vi "NumberDetector.vi"() -> ()   [LabVIEW 2016]
uses:
  <vilib>/Analysis/3filter.llb/Filter Passband Type.ctl
  <vilib>/myRIO/Instrument Drivers/Onboard Devices/Accelerometer/typedefs/Accelerometer Reference.ctl
  <vilib>/myRIO/Common/Instrument Driver Framework/Utilities/typedefs/myRIO Generic Hardware Reference.ctl
  <vilib>/myRIO/Common/Instrument Driver Framework/Utilities/typedefs/Hardware Version Enum.ctl
  <vilib>/myRIO/Common/Instrument Driver Framework/Utilities/typedefs/myRIO v1.0 Reference.ctl
  <vilib>/myRIO/Common/Instrument Driver Framework/Utilities/typedefs/Generic FPGA Reference.ctl
  <vilib>/myRIO/Common/Instrument Driver Framework/myRIO v1.0/Accelerometer/typedefs/Accelerometer Channels List.ctl
  <vilib>/myRIO/Common/Instrument Driver Framework/myRIO v1.0/Accelerometer/typedefs/Accelerometer Channels Enum.ctl
  <vilib>/userdefined/High Color/nirio_resource_hc.ctl
  <vilib>/myRIO/Common/Instrument Driver Framework/Utilities/vis/Is FPGA Ref Available.vi
  <vilib>/myRIO/Common/Instrument Driver Framework/myRIO v1.0/Accelerometer/vis/myRIO v1.1 Open Accelerometer.vi
  <vilib>/myRIO/Instrument Drivers/Onboard Devices/Accelerometer/vis/Read.vi
  <vilib>/Analysis/baseanly.llb/A x Vector.vi
  <vilib>/myRIO/Common/Instrument Driver Framework/Utilities/vis/Validate Channels.vi
  <vilib>/myRIO/Common/Instrument Driver Framework/myRIO v1.0/Accelerometer/vis/myRIO v1.0 Reserve Accelerometer.vi
  <vilib>/myRIO/Common/Instrument Driver Framework/myRIO v1.0/UART/vis/myRIO v1.0 Close UART.vi
  <vilib>/myRIO/Common/Instrument Driver Framework/myRIO v1.0/Resource Manager/vis/myRIO v1.0 Reserve Channel List.vi
  <vilib>/myRIO/Common/Instrument Driver Framework/myRIO v1.0/Accelerometer/vis/myRIO v1.0 Build MUX Configuration Accelerometer.vi
  <vilib>/myRIO/Common/Instrument Driver Framework/myRIO v1.0/Resource Manager/vis/myRIO v1.0 Reserve Channel.vi
  <vilib>/myRIO/Common/Instrument Driver Framework/myRIO v1.0/Resource Manager/vis/myRIO v1.0 Unreserve Channel.vi
  <vilib>/myRIO/Common/Instrument Driver Framework/myRIO v1.0/Resource Manager/vis/myRIO v1.0 Build Mutex Name.vi
  <vilib>/Utility/VariantDataType/GetNumericInfo.vi
  <vilib>/Utility/error.llb/Error Cluster From Error Code.vi
  <vilib>/myRIO/Common/Instrument Driver Framework/myRIO v1.0/myRIO v1.1 Open.vi
  <vilib>/myRIO/Common/Instrument Driver Framework/myRIO v1.0/Accelerometer/vis/myRIO v1.0 Get Scaling Constant Accelerometer.vi
  <vilib>/myRIO/Common/Instrument Driver Framework/Utilities/vis/IO Manager.vi
  <vilib>/myRIO/Common/Instrument Driver Framework/Utilities/vis/Configuration Manager.vi
  <vilib>/myRIO/Common/Instrument Driver Framework/myRIO v1.0/myRIO v1.0 Close.vi
  <vilib>/myRIO/Common/Instrument Driver Framework/myRIO v1.0/Accelerometer/vis/myRIO v1.0 Read Accelerometer.vi
  <vilib>/myRIO/Common/Instrument Driver Framework/Utilities/vis/FPGA Ref Manager.vi
  <vilib>/myRIO/Common/Instrument Driver Framework/myRIO v1.0/myRIO v1.0 Reset FPGA.vi
  <vilib>/myRIO/Common/Instrument Driver Framework/myRIO v1.0/IRQ/vis/myRIO v1.0 IRQ Info FGV.vi
  <vilib>/myRIO/Common/Instrument Driver Framework/myRIO v1.0/IRQ/vis/myRIO v1.0 Timer IRQ Info FGV.vi
  <vilib>/myRIO/Common/Instrument Driver Framework/myRIO v1.0/IRQ/vis/myRIO v1.0 ISR Agent.vi
  <vilib>/myRIO/Express VI/Onboard Devices/Accelerometer/Accelerometer Express VI.xnode
  <vilib>/myRIO/Instrument Drivers/Onboard Devices/Accelerometer/vis/myRIO Accelerometer Open.xnode
  <vilib>/Analysis/NI_AALBase.lvlib
  <vilib>/myRIO/Instrument Drivers/Onboard Devices/Accelerometer/Accelerometer.lvlib
  <vilib>/ptbypt/NI_PtbyPt.lvlib
  <vilib>/myRIO/Instrument Drivers/Utilities/Utilities.lvlib
panel:
  in  "Stop Data Collect 2":bool
  out "Network Ouput Array 3":dbl[][](array[numeric])
  out "Network Ouput Array 2":dbl[][](array[numeric])
  out "Numeric":dbl
  out "Network Ouput Array":dbl[](array[numeric])
  out "Input Data as 2D":dbl[][](array[numeric])
  out "Input Data as 1D":dbl[](array[numeric])
  out "Raw Values":T1(graph) caption="Waveform Chart"
  in  "Stop Data Collect":bool
  out "Pitch and Roll":cluster{"r":dbl, "p":dbl}(graph) caption="Waveform Chart"
  out "?":dbl
  out "error out":errorcluster
  in  "Start Data Collect":bool
  # "Input View"
  # "Output View"
  # "Data Collect Control"
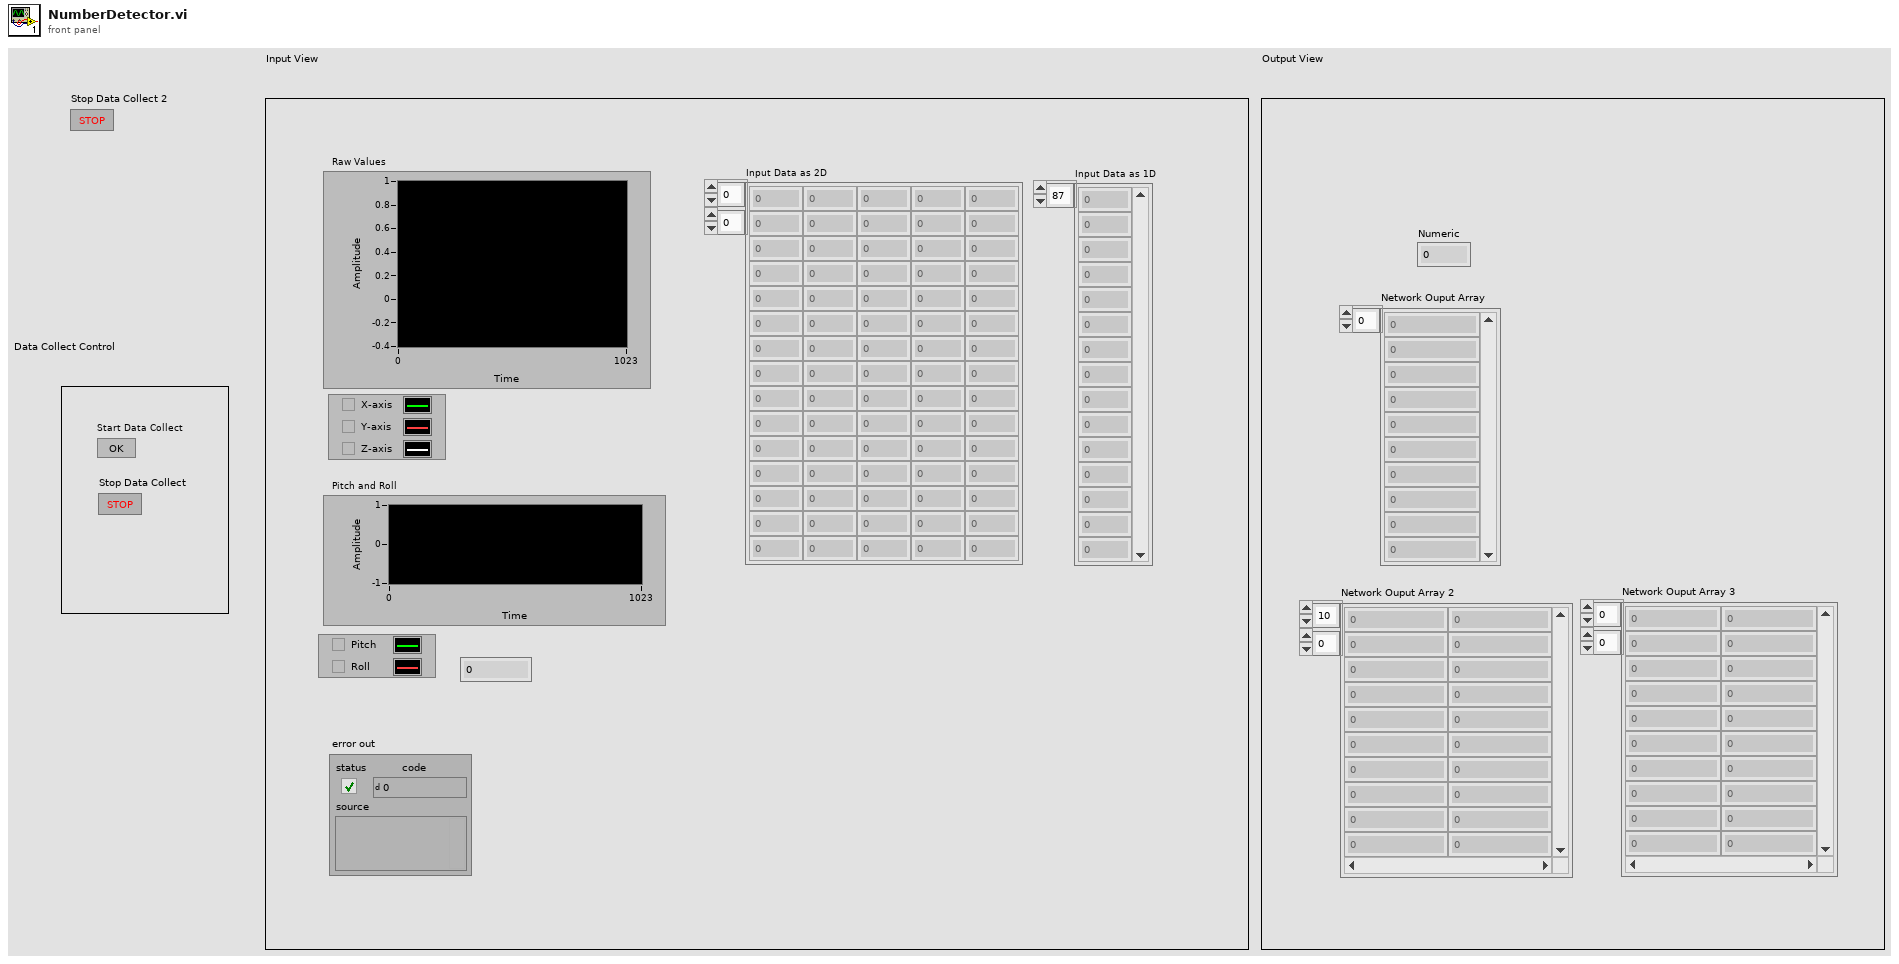
[diagram p1: front panel]
types:
  T1 = cluster{"X-Axis":dbl, "Y-Axis":dbl, "Z-Axis":dbl}
  T2 = typedef "Accelerometer.lvlib/Accelerometer Reference.ctl" = cluster{"myRIO Reference":T3, "Accelerometer Channels List":T7, "LSB Weight":dbl}
  T3 = typedef "myRIO Generic Hardware Reference.ctl" = cluster{"myRIO Model":T4, "myRIO Hardware Reference":T5}
  T4 = typedef "Hardware Version Enum.ctl" = enum16{"Unknown", "myRIO-1900", "myRIO-1950", "roboRIO", "NI ELVIS RIO CM"}
  T5 = typedef "myRIO v1.0 Reference.ctl" = cluster{"Generic FPGA Reference":T6, "Allow multiple opens":bool}
  T6 = typedef "Generic FPGA Reference.ctl" = refnum<k20>
  T7 = typedef "Accelerometer Channels List.ctl" = T8[]
  T8 = typedef "Accelerometer Channels Enum.ctl" = enum16{"Not Connected", "X-Axis", "Y-Axis", "Z-Axis"}
  T9 = typedef "nirio_resource_hc.ctl" = tag
  T10 = typedef "NI_AALBase.lvlib/Filter Passband Type.ctl" = enum32{"Lowpass", "Highpass", "Bandpass", "Bandstop"}
  T11 = cluster{"Filtered x":dbl, "Filtered x":dbl, "Filtered x":dbl}
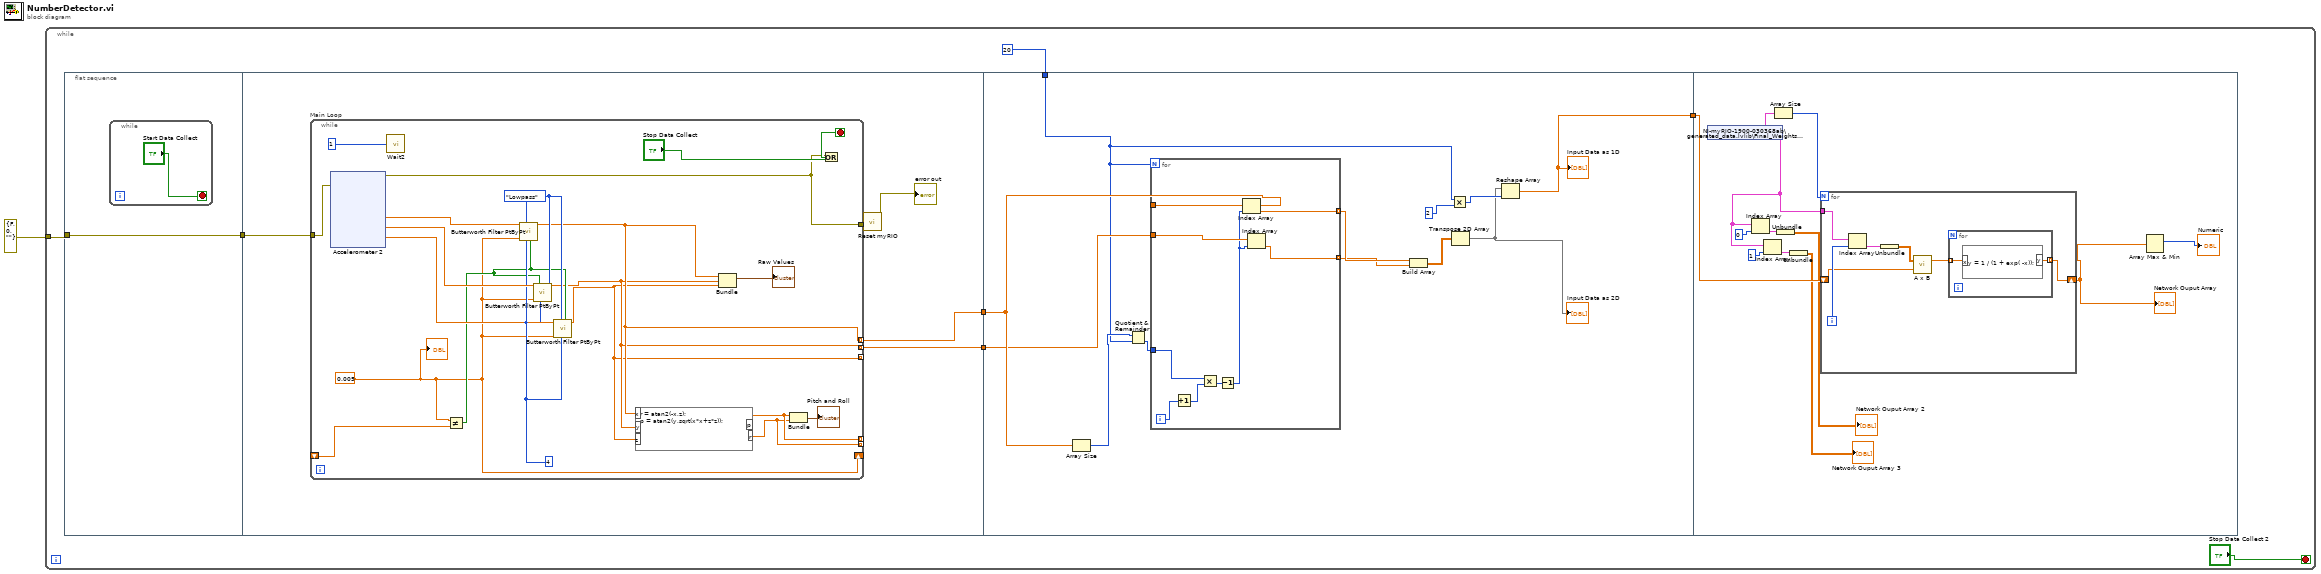
[diagram p0: block diagram]
diagram:
  n1 = while {
    tunnel: errorcluster {"status"=FALSE, "code"=0, "source"=""} ("error in (no error)") -> [w4]
    stop <- "Stop Data Collect 2" stop-if-true
    n2 = flat-sequence {
      tunnel: w4 -> [w9]
      tunnel: [w9] -> w8
      tunnel: [w13] -> w7
      tunnel: w8 -> [w12]
      tunnel: [w11] -> w6
      tunnel: w7 -> [w85]
      tunnel: w6 -> [w83]
      tunnel: 20 -> [w75]
      tunnel: [w76] -> w5
      tunnel: w5 -> [w103]
      frame #0 {
        n3 = while {
          stop <- "Start Data Collect" stop-if-true
        }
      }
      frame #1 {
        n4 = while "Main Loop" {
          tunnel: [w31] -> w15
          tunnel: w12 -> [w32]
          tunnel: [w28] -> _ mode=indexing
          tunnel: [w27] -> _ mode=indexing
          tunnel: [w19] -> w13 mode=indexing
          tunnel: [w18] -> w11 mode=indexing
          tunnel: [w17] -> _ mode=indexing
          shift-right: [w16] -> _
          shift-left: _ -> [w22]
          stop <- w33 stop-if-true
          w16 = 0.005
          w23 = 4
          w26 = Filter_Passband_Type."Lowpass" ("filter type")
          n5 = xnode "Accelerometer 2"("error in (no error)"=w32) -> ("X-Axis"=w20:dbl, "Y-Axis"=w25:dbl, "Z-Axis"=w24:dbl, "error out"=w31:errorcluster)
          n6 = call "Wait2"("Count(mSec)"=1) -> ()  [unwired: 1 out]
          n7 = Not Equal?(x=w16, y=w22) -> (x != y?=w21:bool)
          n8 = call <vilib>:"Butterworth Filter PtByPt.vi"("initialize"=w21, "order"=w23, "filter type"=w26, "low cutoff freq: fl"=w16, "x"=w20) -> ("Filtered x"=w19:dbl)  [unwired: 4 in, 1 out]
          n9 = call <vilib>:"Butterworth Filter PtByPt.vi"("initialize"=w21, "order"=w23, "filter type"=w26, "low cutoff freq: fl"=w16, "x"=w25) -> ("Filtered x"=w18:dbl)  [unwired: 4 in, 1 out]
          n10 = call <vilib>:"Butterworth Filter PtByPt.vi"("initialize"=w21, "order"=w23, "filter type"=w26, "low cutoff freq: fl"=w16, "x"=w24) -> ("Filtered x"=w17:dbl)  [unwired: 4 in, 1 out]
          n11 = formula code="r = atan2(-x,z);\np = atan2(y,sqrt(x*x+z*z));"("y"=w18, "z"=w17, "x"=w19) -> ("p"=w28:dbl, "r"=w27:dbl)
          n12 = Bundle("Filtered x"=w19, "Filtered x"=w18, "Filtered x"=w17) -> (→"Raw Values":T11)  [unwired: 1 in]
          n13 = Bundle("p"=w28, "r"=w27) -> (→"Pitch and Roll":cluster{"p":dbl, "r":dbl})  [unwired: 1 in]
          n14 = Or(x=w31, y="Stop Data Collect") -> (x .or. y?=w33:bool)
          "?" <- w16
        }
        n15 = call <vilib>:"Reset myRIO.vi"("error in (no error)"=w15) -> ("error out"=→"error out":errorcluster)  [unwired: 10 in]
      }
      frame #2 {
        n16 = Array Size(array=w85) -> (size(s)=w86:i32)
        n17 = Quotient & Remainder(x=w86, y=w75) -> (floor(x/y)=w84:i32)  [unwired: 1 out]
        n18 = for {
          N: w75 -> [_]
          tunnel: w85 -> [w92]
          tunnel: w84 -> [w93]
          tunnel: [w91] -> w82 mode=indexing
          tunnel: w83 -> [w90]
          tunnel: [w89] -> w81 mode=indexing
          i -> [w94]
          n19 = Increment(x=w94) -> (x+1=w95:i32)
          n20 = Multiply(x=w93, y=w95) -> (x*y=w88:i32)
          n21 = Decrement(x=w88) -> (x-1=w87:i32)
          n22 = Index Array(array=w92, index=w87) -> (element=w91:dbl)
          n23 = Index Array(array=w90, index=w87) -> (element=w89:dbl)
        }
        n24 = Build Array(w82, w81) -> (w80:dbl[][])
        n25 = Multiply(x=w75, y=2) -> (x*y=w78:i32)
        n26 = Transpose 2D Array(2D array=w80) -> (transposed array=w77:dbl[][])
        "Input Data as 2D" <- w77
        n27 = Reshape Array(w77, w78) -> (w76:dbl[])
        "Input Data as 1D" <- w76
      }
      frame #3 {
        n28 = shared-variable "NI-myRIO-1900-030368ab\\generated_data.lvlib\\Final_Weights_2"() -> (w98:cluster{dbl[][]}[])  [unwired: 1 in, 1 out]
        n29 = Index Array(array=w98, index=0) -> (element=w102:cluster{dbl[][]})
        n30 = Index Array(array=w98, index=1) -> (element=w100:cluster{dbl[][]})
        n31 = Array Size(array=w98) -> (size(s)=w106:i32)
        n32 = Unbundle(w102) -> (→"Network Ouput Array 2":dbl[][])
        n33 = Unbundle(w100) -> (→"Network Ouput Array 3":dbl[][])
        n34 = for {
          N: w106 -> [_]
          tunnel: w98 -> [w107]
          shift-right: [w110] -> w105
          shift-left: w103 -> [w108]
          i -> [w112]
          n35 = Index Array(array=w107, index=w112) -> (element=w113:cluster{dbl[][]})
          n36 = Unbundle(w113) -> (w109:dbl[][])
          n37 = call-poly <vilib>:"A x B.vi"("Vector"=w108, "A"=w109) -> ("A x Vector"=w111:dbl[])  [unwired: 1 out]
          n38 = for {
            tunnel: w111 -> [w115] mode=indexing
            tunnel: [w114] -> w110 mode=indexing
            n39 = formula code="y = 1 / (1 + exp( -x));"("x"=w115) -> ("y"=w114:dbl)
          }
        }
        "Network Ouput Array" <- w105
        n40 = Array Max & Min(array=w105) -> (max index (indices)=→"Numeric":i32)  [unwired: 3 out]
      }
    }
  }
